vi "Globals.vi"() -> ()   [LabVIEW 2017]
panel:
  out "Version":string="1.0.0"
  in  "NumOfConnections":u32
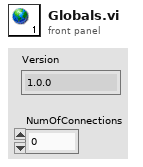
[diagram p1: front panel]
diagram:
